vi "Save calib config.vi"(8 "Error In":errorcluster, 11 "UI data in":T1={"GPIB Addresses"={"GPIB Motor"=2, "GPIB Laser"="3"}, "Beam size"={"BeamX"=0.0, "BeamY"=0.0, "Beam Overlap"=0.0}, "Motor speed"={"Xspeed"=0.0, " Yspeed"=0.0}, "Laser parameters"={"Thyratron Bias"=20.0, "Frequency"=0, "Shots/Point"=0.0}, "Irradiation points"={"X1"=0.0, "Y1"=0.0, "X2"=0.0, "Y2"=0.0}, "Calibration Point"={"Xcalib"=0.0, "Ycalib"=0.0}} {"Laser parameters"."Frequency" format="%.0fHz"; "Laser parameters"."Thyratron Bias" format="%#_gkV"}) -> (0 "Error Out":errorcluster, 3 "UI data out":T1={"GPIB Addresses"={"GPIB Motor"=2, "GPIB Laser"="3"}, "Beam size"={"BeamX"=0.0, "BeamY"=0.0, "Beam Overlap"=0.0}, "Motor speed"={"Xspeed"=0.0, " Yspeed"=0.0}, "Laser parameters"={"Thyratron Bias"=20.0, "Frequency"=0, "Shots/Point"=0.0}, "Irradiation points"={"X1"=0.0, "Y1"=0.0, "X2"=0.0, "Y2"=0.0}, "Calibration Point"={"Xcalib"=0.0, "Ycalib"=0.0}} {"Laser parameters"."Frequency" format="%.0fHz"; "Laser parameters"."Thyratron Bias" format="%#_gkV"})   [LabVIEW 2014]
uses:
  Typedef/UI data.ctl
  <vilib>/Utility/config.llb/Write Key (Double).vi
  <vilib>/Utility/config.llb/NI_LVConfig.lvlib
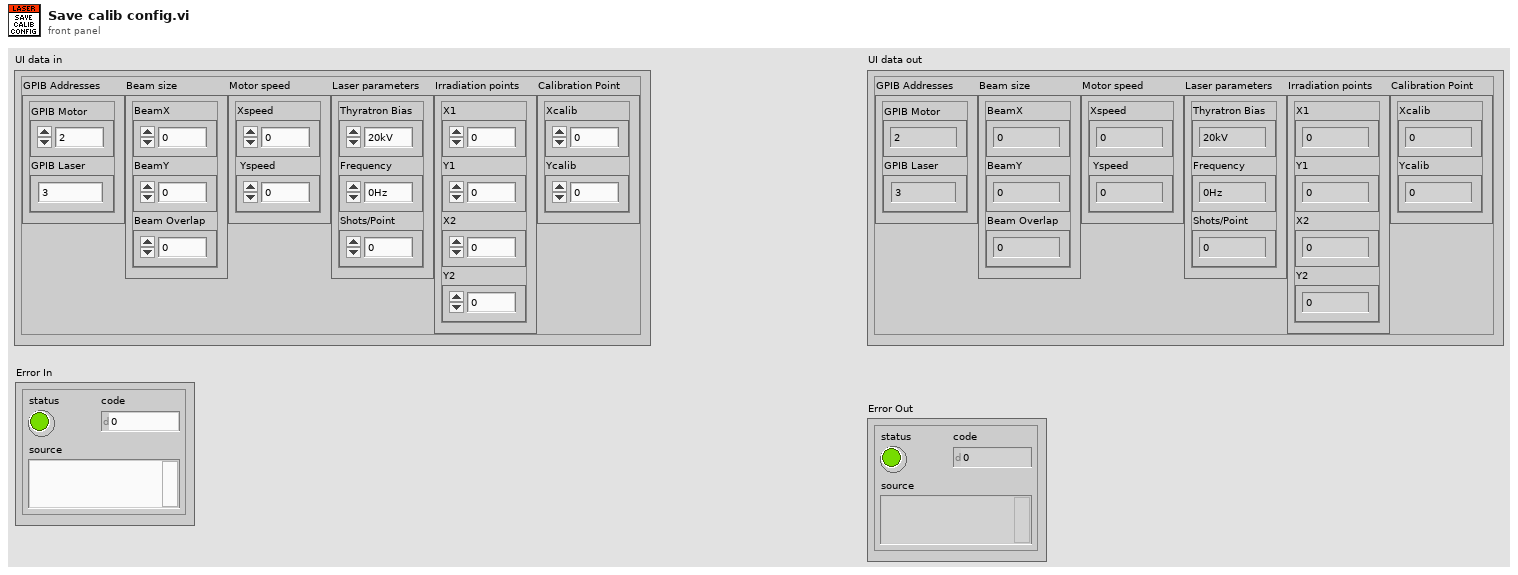
[diagram p1: front panel]
types:
  T1 = typedef "UI data.ctl" = cluster{"GPIB Addresses":cluster{"GPIB Motor":i16, "GPIB Laser":string}, "Beam size":cluster{"BeamX":dbl, "BeamY":dbl, "Beam Overlap":dbl}, "Motor speed":cluster{"Xspeed":dbl, " Yspeed":dbl}, "Laser parameters":cluster{"Thyratron Bias":dbl, "Frequency":u16, "Shots/Point":dbl}, "Irradiation points":cluster{"X1":dbl, "Y1":dbl, "X2":dbl, "Y2":dbl}, "Calibration Point":cluster{"Xcalib":dbl, "Ycalib":dbl}}
  T2 = typedef "NI_LVConfig.lvlib/Config Data RefNum.ctl" = refnum<k1>
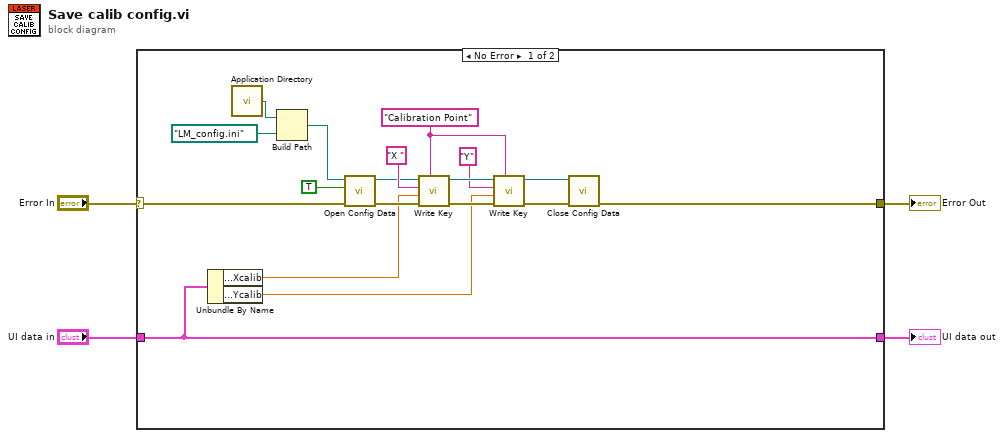
[diagram p0: block diagram]
diagram:
  n1 = case shown="No Error" "Error In" {
    selector: "Error In" -> [w19 w24]
    tunnel: [w6 w24] -> w3
    tunnel: "UI data in" -> [w5 w23]
    tunnel: [w5 w23] -> w1
    frame No Error {
      w10 = "Calibration Point" ("section")
      n2 = Unbundle By Name(w5) -> ("Calibration Point.Xcalib"=w16:dbl, "Calibration Point.Ycalib"=w9:dbl)
      n3 = call <vilib>:"Application Directory.vi"() -> ("Application Directory"=w22:path)
      n4 = Build Path(base path=w22, name or relative path=path "LM_config.ini" ("default name")) -> (appended path=w20:path)
      n5 = call <vilib>:"Open Config Data.vi"("error in (no error)"=w19, "create file if necessary (T)"=TRUE, "configuration file path"=w20) -> ("error out"=w17:errorcluster, "refnum"=w14:T2)  [unwired: 6 in, 1 out]
      n6 = call-poly <vilib>:"Write Key.vi"("section"=w10, "error in (no error)"=w17, "value"=w16, "key"="X ", "refnum"=w14) -> ("error out"=w12:errorcluster, "refnum out"=w13:T2)  [unwired: 4 in, 1 out]
      n7 = call-poly <vilib>:"Write Key.vi"("section"=w10, "error in (no error)"=w12, "value"=w9, "key"="Y", "refnum"=w13) -> ("error out"=w8:errorcluster, "refnum out"=w7:T2)  [unwired: 4 in, 1 out]
      n8 = call <vilib>:"Close Config Data.vi"("error in (no error)"=w8, "refnum"=w7) -> ("error out"=w6:errorcluster)  [unwired: 8 in, 1 out]
    }
    frame Error {
    }
  }
  "Error Out" <- w3
  "UI data out" <- w1
